vi "SwitchBoard_ReadEnvSensors.vi"(8 "error in":errorcluster, 11 "Handle":u32) -> (0 "error out":errorcluster, 1 "Matrix humidity":dbl, 2 "Matrix temperature":dbl, 3 "Handle out":u32, 7 "current time":timestamp)   [LabVIEW 2016]
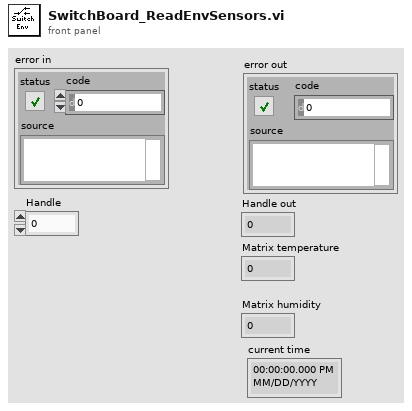
[diagram p1: front panel]
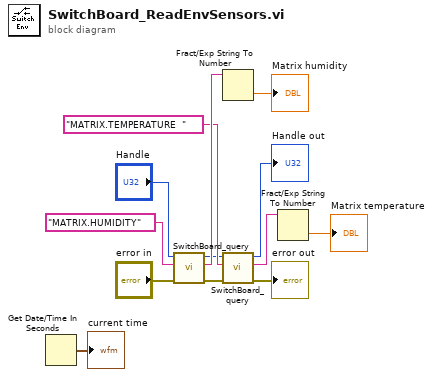
[diagram p0: block diagram]
diagram:
  n1 = Get Date/Time In Seconds() -> (seconds since 1Jan1904=→"current time":timestamp)
  n2 = call "SwitchBoard_query.vi"("error in"="error in", "Buffer"="MATRIX.HUMIDITY" ("string"), "Handle"="Handle") -> ("error out"=w1:errorcluster, "Read Buffer Out"=w10:string, "Handle"=w6:u32)  [unwired: 6 in]
  n3 = Fract/Exp String To Number(string=w10) -> (number=→"Matrix humidity":dbl)  [unwired: 3 in, 1 out]
  n4 = call "SwitchBoard_query.vi"("error in"=w1, "Buffer"="MATRIX.TEMPERATURE  " ("string"), "Handle"=w6) -> ("error out"=→"error out":errorcluster, "Read Buffer Out"=w5:string, "Handle"=→"Handle out":u32)  [unwired: 6 in]
  n5 = Fract/Exp String To Number(string=w5) -> (number=→"Matrix temperature":dbl)  [unwired: 3 in, 1 out]
